vi "Demo.vi"() -> ()   [LabVIEW 2020]
doc: "This will prevent the system from sleeping when run and will prevent the screen-saver from turning on when the mouse is hovered over the 'Keep Screen On' button."
uses:
  Power Availabilty Requests/Type Defs/Power Request Type.ctl
  Power Requests.lvlib
panel:
  in  "stop":bool
  in  "Keep Screen On":bool
  # "Overview: This will prevent the system from sleeping when run and will prevent the screen-saver from turning on when the mouse is hovered over the Keep Screen On button.\nRequirements: LabVIEW 2012 (or compatible)\nInstructions: \n1. Run this VI"
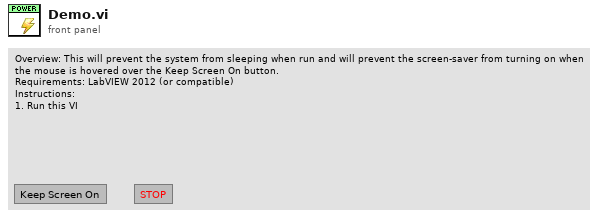
[diagram p1: front panel]
types:
  T1 = typedef "Power Requests.lvlib/Power Request Type.ctl" = enum32{"Power Request Display Required", "Power Request System Required", "Power Request Away Mode Required", "Power Request Execution Required"}
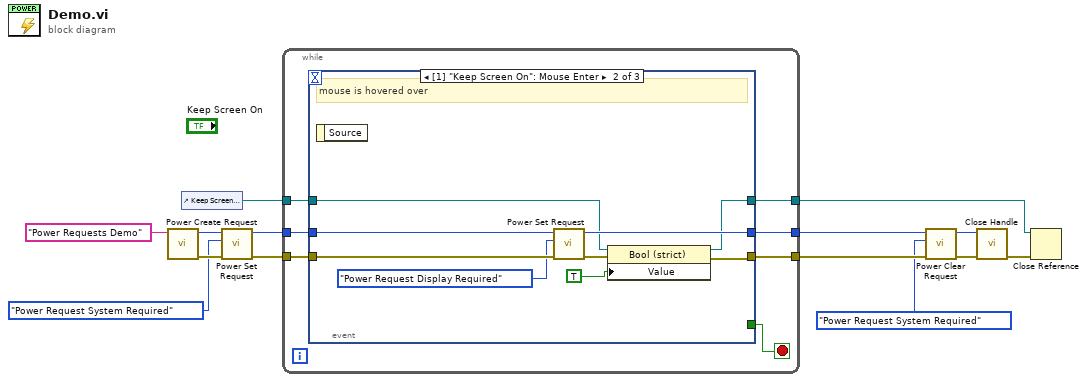
[diagram p0: block diagram]
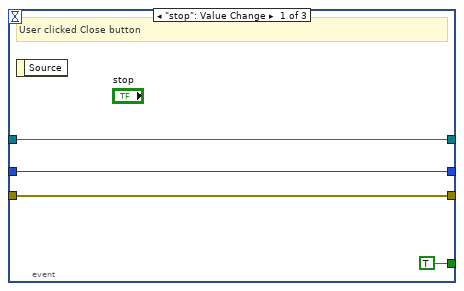
[diagram p2: hidden frame]
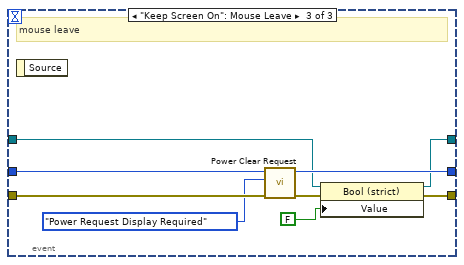
[diagram p3: hidden frame]
diagram:
  n1 = call "Power Create Request.vi"("Simple Reason String"="Power Requests Demo") -> ("error out"=w14:errorcluster, "Handle"=w13:i64)  [unwired: 9 in]
  n2 = control-ref of="Keep Screen On"() -> (w3:refnum<vi>)
  n3 = call "Power Set Request.vi"("error in (no error)"=w14, "Power Request Type"=Power_Request_Type."Power Request System Required", "Handle in"=w13) -> ("error out"=w12:errorcluster, "Handle out"=w5:u32)  [unwired: 6 in, 1 out]
  n4 = while {
    tunnel: w12 -> [w20]
    tunnel: [w19] -> w11
    tunnel: w5 -> [w18]
    tunnel: [w17] -> w4
    tunnel: w3 -> [w16]
    tunnel: [w15] -> w1
    stop <- w21 stop-if-true
    n5 = event shown="[1] \"Keep Screen On\": Mouse Enter" {
      selector: _ -> [_ _ _]
      dyn-events: _ -> [_ _ _]
      timeout: _ -> [_ _ _]
      tunnel: [TRUE _ _] -> w21
      tunnel: w20 -> [w25 w32 w43]
      tunnel: [w25 w29 w38] -> w19
      tunnel: w18 -> [w24 w34 w42]
      tunnel: [w24 w33 w41] -> w17
      tunnel: w16 -> [w23 w28 w37]
      tunnel: [w23 w27 w36] -> w15
      event "stop": Value Change {
        # "User clicked Close button"
        n6 = event-data() -> ()  [unwired: 1 in, 1 out]
      }
      event "Keep Screen On": Mouse Enter {
        # "mouse is hovered over"
        n7 = event-data() -> ()  [unwired: 1 in, 1 out]
        n8 = call "Power Set Request.vi"("error in (no error)"=w32, "Power Request Type"=Power_Request_Type."Power Request Display Required", "Handle in"=w34) -> ("error out"=w30:errorcluster, "Handle out"=w33:u32)  [unwired: 6 in, 1 out]
        n9 = property class="Bool (strict)"(reference=w28, error in=w30, "Value"=TRUE) -> (reference out=w27:refnum<vi>, error out=w29:errorcluster)
      }
      event "Keep Screen On": Mouse Leave {
        # "mouse leave"
        n10 = event-data() -> ()  [unwired: 1 in, 1 out]
        n11 = call "Power Clear Request.vi"("error in (no error)"=w43, "Power Request Type"=Power_Request_Type."Power Request Display Required", "Handle in"=w42) -> ("error out"=w39:errorcluster, "Handle out"=w41:u32)  [unwired: 6 in, 1 out]
        n12 = property class="Bool (strict)"(reference=w37, error in=w39, "Value"=FALSE) -> (reference out=w36:refnum<vi>, error out=w38:errorcluster)
      }
    }
  }
  n13 = call "Power Clear Request.vi"("error in (no error)"=w11, "Power Request Type"=Power_Request_Type."Power Request System Required", "Handle in"=w4) -> ("error out"=w10:errorcluster, "Handle out"=w9:u32)  [unwired: 6 in, 1 out]
  n14 = call "Close Handle.vi"("error in (no error)"=w10, "Handle"=w9) -> ("error out"=w2:errorcluster)  [unwired: 8 in, 1 out]
  n15 = Close Reference(reference=w1, error in (no error)=w2) -> ()  [unwired: 1 out]
